vi "Register for Events.vi"(8 "error in (no error)":errorcluster, 11 "Process State":refnum<data-value>) -> (0 "error out":errorcluster, 2 "Event Registration Refnum":refnum<event-registration>, 3 "Process State":refnum<data-value>)   [LabVIEW 2022 SP3, in "Process State Data.lvclass"]
uses:
  Process State Data.lvclass
  Process State Data.lvclass/Process State Data.ctl
  Events.ctl
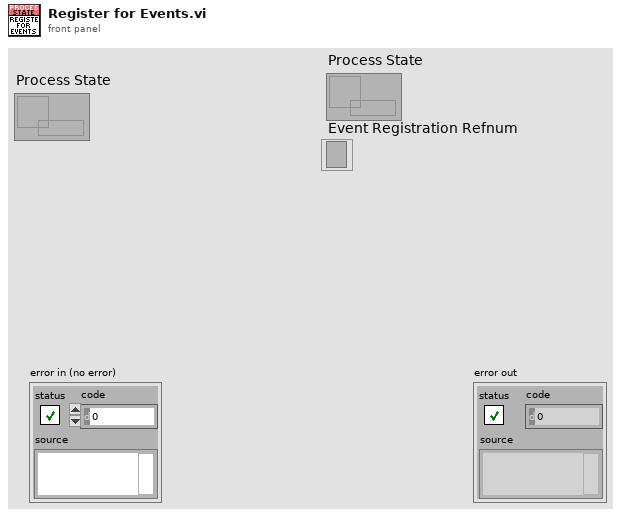
[diagram p1: front panel]
types:
  T1 = typedef "Process State Data.lvclass/Events.ctl" = cluster{"Busy":refnum<user-event>, "Abort":refnum<user-event>, "Proccess Error":refnum<user-event>}
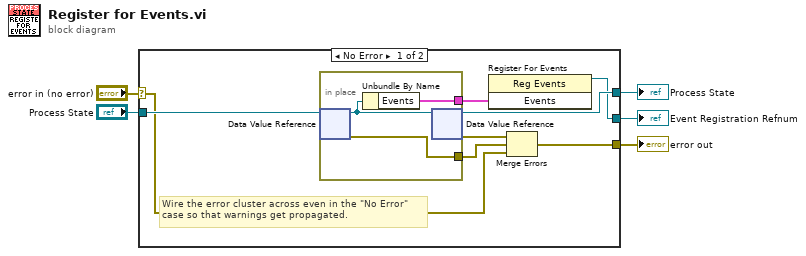
[diagram p0: block diagram]
diagram:
  n1 = case shown="No Error" "error in (no error)" {
    selector: "error in (no error)" -> [w9 w17]
    tunnel: [w8 w17] -> w4
    tunnel: "Process State" -> [w13 _]
    tunnel: [w12 _] -> w2
    tunnel: [w6 _] -> w1
    frame No Error {
      # "Wire the error cluster across even in the \"No Error\"\ncase so that warnings get propagated."
      n2 = in-place {
        in-place-border: [w16] -> w7
        in-place-border: [w14] -> w10
        n3 = in-place-dvr #1(w13) -> (w15:refnum<class "Process State Data.lvclass">, w14:errorcluster)
        n4 = Unbundle By Name(w15) -> ("Events"=w16:T1)
        n5 = in-place-dvr #1(w15) -> (w12:refnum<data-value>, w11:errorcluster)
      }
      n6 = register-events(w7) -> (reference out=w6:refnum<event-registration>)  [unwired: 2 in, 1 out]
      n7 = Merge Errors(w11, w10, w9) -> (w8:errorcluster)
    }
    frame Error {
    }
  }
  "error out" <- w4
  "Process State" <- w2
  "Event Registration Refnum" <- w1
